vi "remove missing files.vi"(11 "cache in":T1) -> (3 "cache out":T1)   [LabVIEW 2013, in "PL_class cache.lvlib"]
uses:
  PL_class cache.lvlib
  cache definition.ctl
  cache search configuration.ctl
  cached class information.ctl
  target class metadata.ctl
  class metadata.ctl
  <vilib>/NI/Tag Bus Module Framework/root configuration/Target Types.ctl
  <vilib>/NI/Tag Bus Module Framework/root configuration/TBM configuration.lvclass
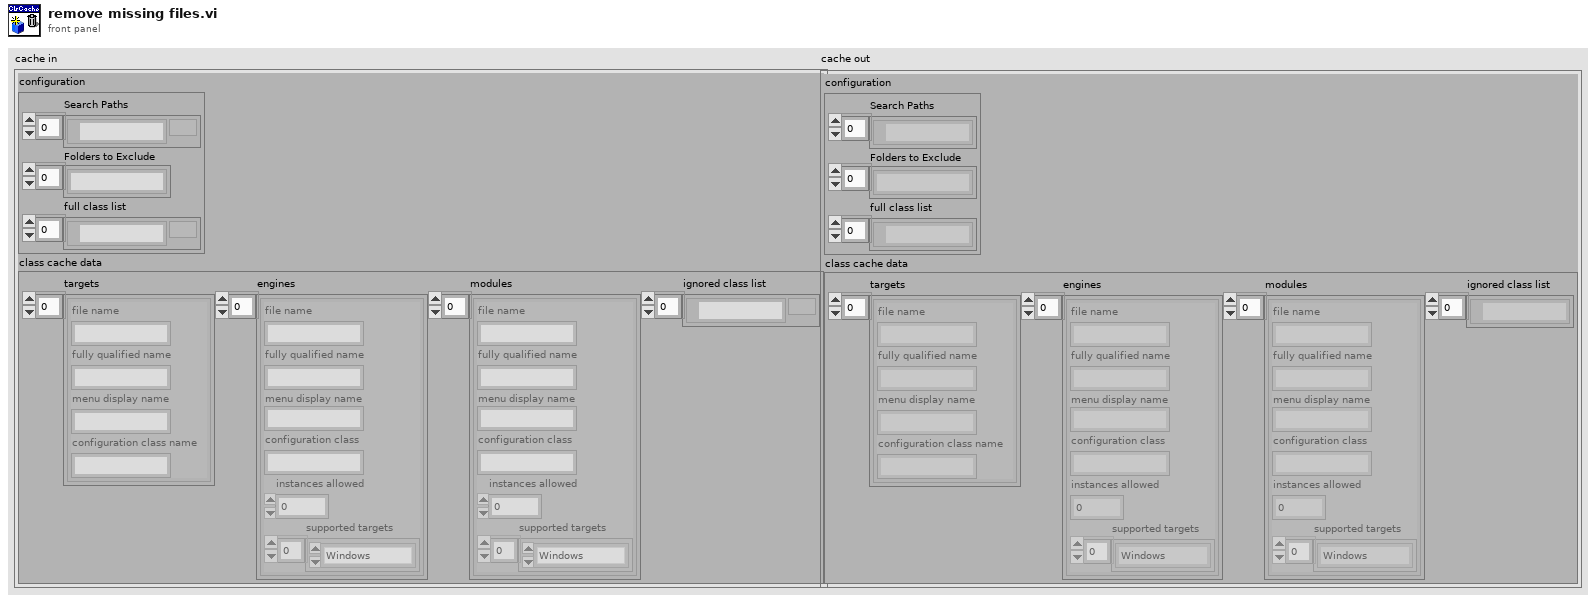
[diagram p1: front panel]
types:
  T1 = typedef "PL_class cache.lvlib/cache definition.ctl" = cluster{"configuration":T2, "class cache data":T3}
  T2 = typedef "PL_class cache.lvlib/cache search configuration.ctl" = cluster{"Search Paths":path[], "Folders to Exclude":string[], "full class list":path[]}
  T3 = typedef "PL_class cache.lvlib/cached class information.ctl" = cluster{"targets":T4[], "engines":T5[], "modules":T5[], "ignored class list":path[]}
  T4 = typedef "PL_class cache.lvlib/target class metadata.ctl" = cluster{"file name":string, "fully qualified name":string, "menu display name":string, "configuration class name":string}
  T5 = typedef "PL_class cache.lvlib/class metadata.ctl" = cluster{"file name":string, "fully qualified name":string, "menu display name":string, "configuration class":string, "instances allowed":i32, "supported targets":T6[]}
  T6 = typedef "TBM configuration.lvclass/Target Types.ctl" = enum16{"Windows", "Mac", "Linux", "Linux RT ARM", "VxWorks", "Pharlap", "Other", "Linux RT x64"}
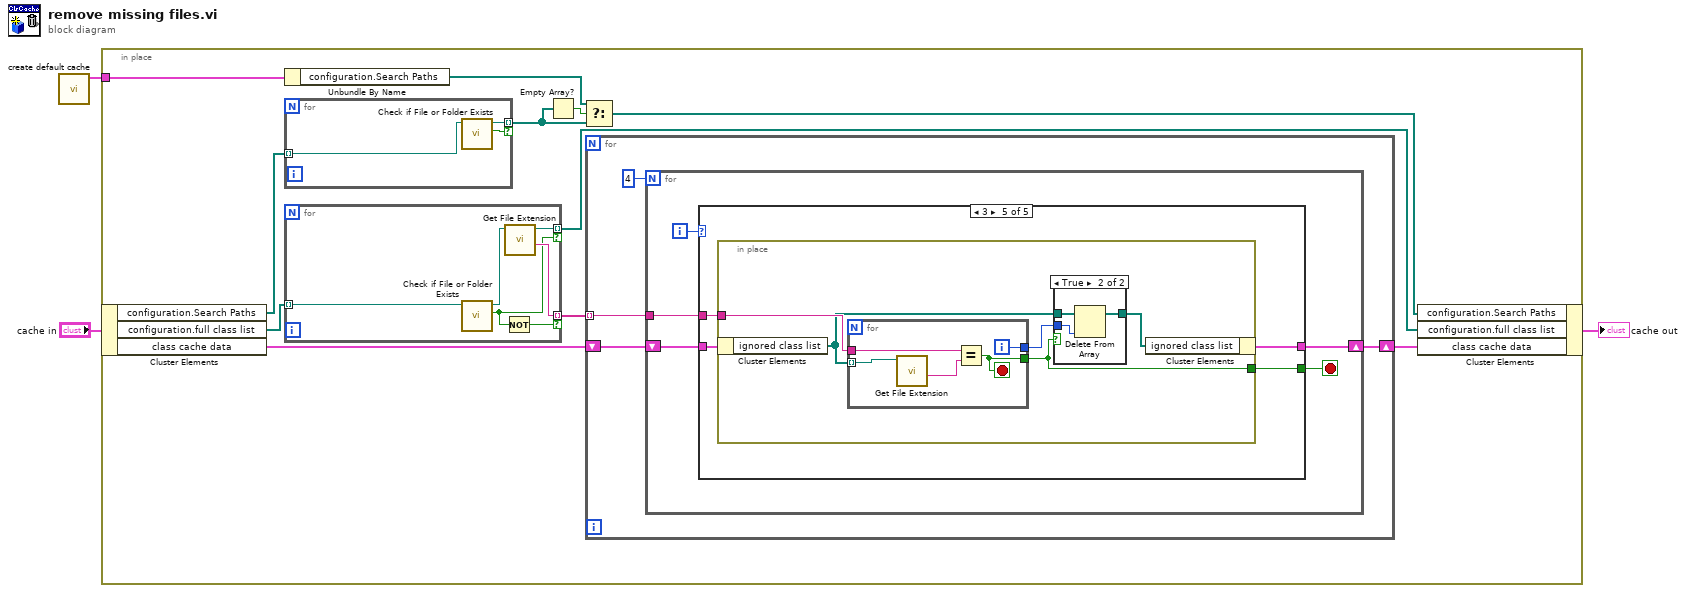
[diagram p0: block diagram]
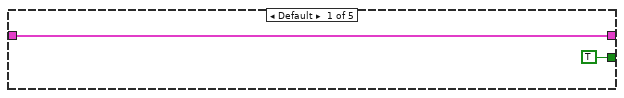
[diagram p2: hidden frame]
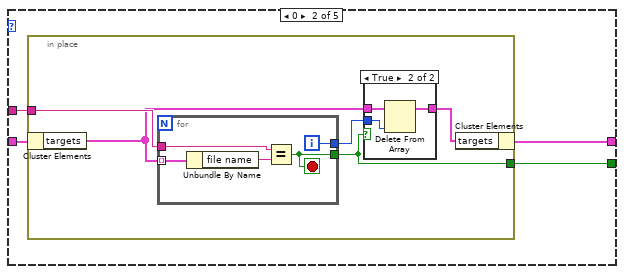
[diagram p3: hidden frame]
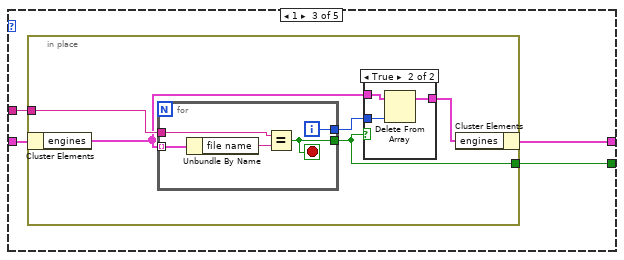
[diagram p5: hidden frame]
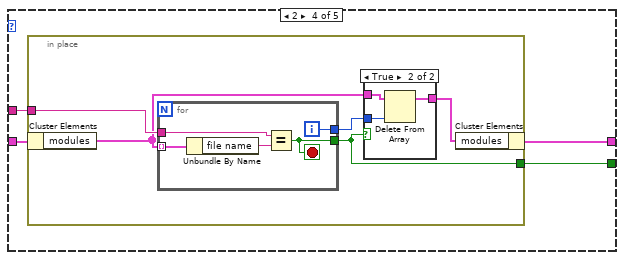
[diagram p7: hidden frame]
diagram:
  n1 = call "create default cache.vi"() -> ("cache"=w2:T1)  [unwired: 11 in]
  n2 = in-place {
    in-place-border: w2 -> [w14]
    n3 = in-place-cluster #1("cache in") -> ("configuration.Search Paths"=w13:path[], "configuration.full class list"=w8:path[], "class cache data"=w5:T3)
    n4 = Unbundle By Name(w14) -> ("configuration.Search Paths"=w11:path[])
    n5 = for {
      tunnel: w13 -> [w106] mode=indexing
      tunnel: [w105] -> w10 mode=indexing if=w104
      n6 = call <vilib>:"Check if File or Folder Exists.vi"("path"=w106) -> ("file or folder exists?"=w104:bool, "dup path"=w105:path)  [unwired: 8 in, 1 out]
    }
    n7 = for {
      tunnel: w8 -> [w103] mode=indexing
      tunnel: [w101] -> w7 mode=indexing if=w99
      tunnel: [w100] -> w6 mode=indexing if=w98
      n8 = call <vilib>:"Check if File or Folder Exists.vi"("path"=w103) -> ("file or folder exists?"=w99:bool, "dup path"=w102:path)  [unwired: 8 in, 1 out]
      n9 = Not(x=w99) -> (.not. x?=w98:bool)
      n10 = call <vilib>:"Get File Extension.vi"("file"=w102) -> ("filename without extension"=w100:string, "dup file"=w101:path)  [unwired: 7 in, 2 out]
    }
    n11 = Empty Array?(array=w10) -> (empty?=w12:bool)
    n12 = Select(t=w11, s=w12, f=w10) -> (s? t:f=w9:path[])
    n13 = for {
      tunnel: w6 -> [w17] mode=indexing
      shift-right: [w15] -> w4
      shift-left: w5 -> [w16]
      n14 = for {
        N: 4 ("Numeric") -> [_]
        tunnel: w17 -> [w19]
        shift-right: [w21] -> w15
        shift-left: w16 -> [w22]
        i -> [w23]
        stop <- w20 stop-if-true
        n15 = case shown="3" w23 {
          tunnel: w22 -> [w25 w29 w47 w65 w83]
          tunnel: [w25 w28 w46 w64 w82] -> w21
          tunnel: [TRUE w26 w44 w62 w80] -> w20
          tunnel: w19 -> [_ w27 w45 w63 w81]
          frame Default {
          }
          frame 0 {
            n16 = in-place {
              in-place-border: w27 -> [w34]
              in-place-border: [w30] -> w26
              n17 = in-place-cluster #2(w29) -> ("targets"=w32:T4[])
              n18 = for {
                tunnel: w32 -> [w43] mode=indexing
                tunnel: w34 -> [w41]
                tunnel: [w40] -> w30
                tunnel: [w39] -> w31
                i -> [w39]
                stop <- w40 stop-if-true
                n19 = Unbundle By Name(w43) -> ("file name"=w42:string)
                n20 = Equal?(x=w41, y=w42) -> (x = y?=w40:bool)
              }
              n21 = case shown="True" w30 {
                tunnel: [w35 w37] -> w33
                tunnel: w32 -> [w35 w38]
                tunnel: w31 -> [_ w36]
                frame False {
                }
                frame True {
                  n22 = Delete From Array(array=w38, index=w36) -> (array with subset deleted=w37:T4[])  [unwired: 1 in, 1 out]
                }
              }
              n23 = in-place-cluster #2("targets"=w33) -> (w28:T3)
            }
          }
          frame 1 {
            n24 = in-place {
              in-place-border: w45 -> [w52]
              in-place-border: [w48] -> w44
              n25 = in-place-cluster #3(w47) -> ("engines"=w50:T5[])
              n26 = for {
                tunnel: w50 -> [w61] mode=indexing
                tunnel: w52 -> [w59]
                tunnel: [w58] -> w48
                tunnel: [w57] -> w49
                i -> [w57]
                stop <- w58 stop-if-true
                n27 = Unbundle By Name(w61) -> ("file name"=w60:string)
                n28 = Equal?(x=w59, y=w60) -> (x = y?=w58:bool)
              }
              n29 = case shown="True" w48 {
                tunnel: [w53 w55] -> w51
                tunnel: w50 -> [w53 w56]
                tunnel: w49 -> [_ w54]
                frame False {
                }
                frame True {
                  n30 = Delete From Array(array=w56, index=w54) -> (array with subset deleted=w55:T5[])  [unwired: 1 in, 1 out]
                }
              }
              n31 = in-place-cluster #3("engines"=w51) -> (w46:T3)
            }
          }
          frame 2 {
            n32 = in-place {
              in-place-border: w63 -> [w70]
              in-place-border: [w66] -> w62
              n33 = in-place-cluster #4(w65) -> ("modules"=w68:T5[])
              n34 = for {
                tunnel: w68 -> [w79] mode=indexing
                tunnel: w70 -> [w77]
                tunnel: [w76] -> w66
                tunnel: [w75] -> w67
                i -> [w75]
                stop <- w76 stop-if-true
                n35 = Unbundle By Name(w79) -> ("file name"=w78:string)
                n36 = Equal?(x=w77, y=w78) -> (x = y?=w76:bool)
              }
              n37 = case shown="True" w66 {
                tunnel: [w71 w73] -> w69
                tunnel: w68 -> [w71 w74]
                tunnel: w67 -> [_ w72]
                frame False {
                }
                frame True {
                  n38 = Delete From Array(array=w74, index=w72) -> (array with subset deleted=w73:T5[])  [unwired: 1 in, 1 out]
                }
              }
              n39 = in-place-cluster #4("modules"=w69) -> (w64:T3)
            }
          }
          frame 3 {
            n40 = in-place {
              in-place-border: w81 -> [w88]
              in-place-border: [w84] -> w80
              n41 = in-place-cluster #5(w83) -> ("ignored class list"=w86:path[])
              n42 = for {
                tunnel: w86 -> [w93] mode=indexing
                tunnel: w88 -> [w97]
                tunnel: [w96] -> w84
                tunnel: [w95] -> w85
                i -> [w95]
                stop <- w96 stop-if-true
                n43 = call <vilib>:"Get File Extension.vi"("file"=w93) -> ("filename without extension"=w94:string)  [unwired: 7 in, 3 out]
                n44 = Equal?(x=w97, y=w94) -> (x = y?=w96:bool)
              }
              n45 = case shown="True" w84 {
                tunnel: [w89 w91] -> w87
                tunnel: w86 -> [w89 w92]
                tunnel: w85 -> [_ w90]
                frame False {
                }
                frame True {
                  n46 = Delete From Array(array=w92, index=w90) -> (array with subset deleted=w91:path[])  [unwired: 1 in, 1 out]
                }
              }
              n47 = in-place-cluster #5("ignored class list"=w87) -> (w82:T3)
            }
          }
        }
      }
    }
    n48 = in-place-cluster #1("configuration.Search Paths"=w9, "configuration.full class list"=w7, "class cache data"=w4) -> (→"cache out":T1)
  }
